vi "IsRefnum.vi"(8 "error in":errorcluster, 11 "UserComment in":refnum<class "UserComment.lvclass">) -> (0 "error out":errorcluster, 2 "IsRefnum":bool, 3 "UserComment out":refnum<class "UserComment.lvclass">)   [LabVIEW 2021, in "ProligentXMLGenerator.lvlib" / "UserComment.lvclass"]
doc: "Returns TRUE if the passed object is valid."
uses:
  UserComment.lvclass
  UserComment.lvclass/UserComment.ctl
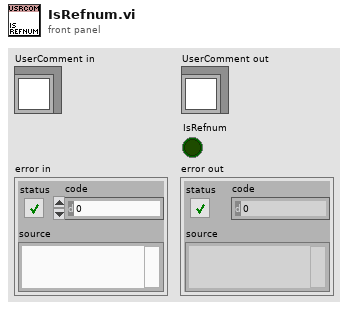
[diagram p1: front panel]
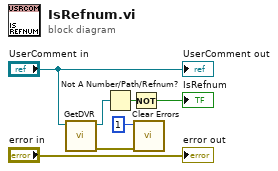
[diagram p0: block diagram]
diagram:
  n1 = call "GetDVR.vi"("UserComment"="UserComment in") -> ("error out"=w1:errorcluster, "DVRReference"=w4:refnum<data-value>)  [unwired: 9 in]
  n2 = Not A Number/Path/Refnum?(number/path/refnum=w4) -> (NaN/Path/Refnum?=w5:bool)
  n3 = Not(x=w5) -> (.not. x?=→"IsRefnum":bool)
  n4 = call <vilib>:"Clear Errors.vi"("error in (no error)"=w1, "specific error code to clear (0: all)"=1) -> ()  [unwired: 4 in, 2 out]
  "error out" <- "error in"
  "UserComment out" <- "UserComment in"
